vi "myo_test.vi"() -> ()   [LabVIEW 2013]
uses:
  <vilib>/BLE/type_def/connection_status_bundle.ctl
  <vilib>/BLE/type_def/address_type.ctl
  <vilib>/BLE/ble_functions/ble_write_by_service_characteristic_uint16.vi
panel:
  out "element":u8
  out "8bit integer 2":i8[][](array[numeric])
  out "8bit integer":u8[][](array[numeric])
  in  "Address Type":T1=1 items=["Public", "Random"]
  out "Readings":i32
  in  "stop":bool
  out "Handle table":string[][](array[string])
  out "Connection Status":T2={"MAC Address"="", "cnx handle"=0, "cnx flags"=0, "Address Type"=125, "Connection Interval (ms)"=125, "Timeout(ms)"=125, "Latency"=0, "bonding handle"=0} {"Address Type" items=["Public", "Random"]}
  out "Scanning":bool
  in  "Continue":bool
  in  "MAC Address":string
  in  "COM Bluegiga in":refnum<visa-resource-name>="COM13"
  out "Devices":string[][](array[string])
  out "BLED112 Dongle Info":string
  # "DISCOVER"
  # "CONNECT"
  # "Introduce the MAC Address of the device you want to connect and click in the CONTINUE button"
  # "READING"
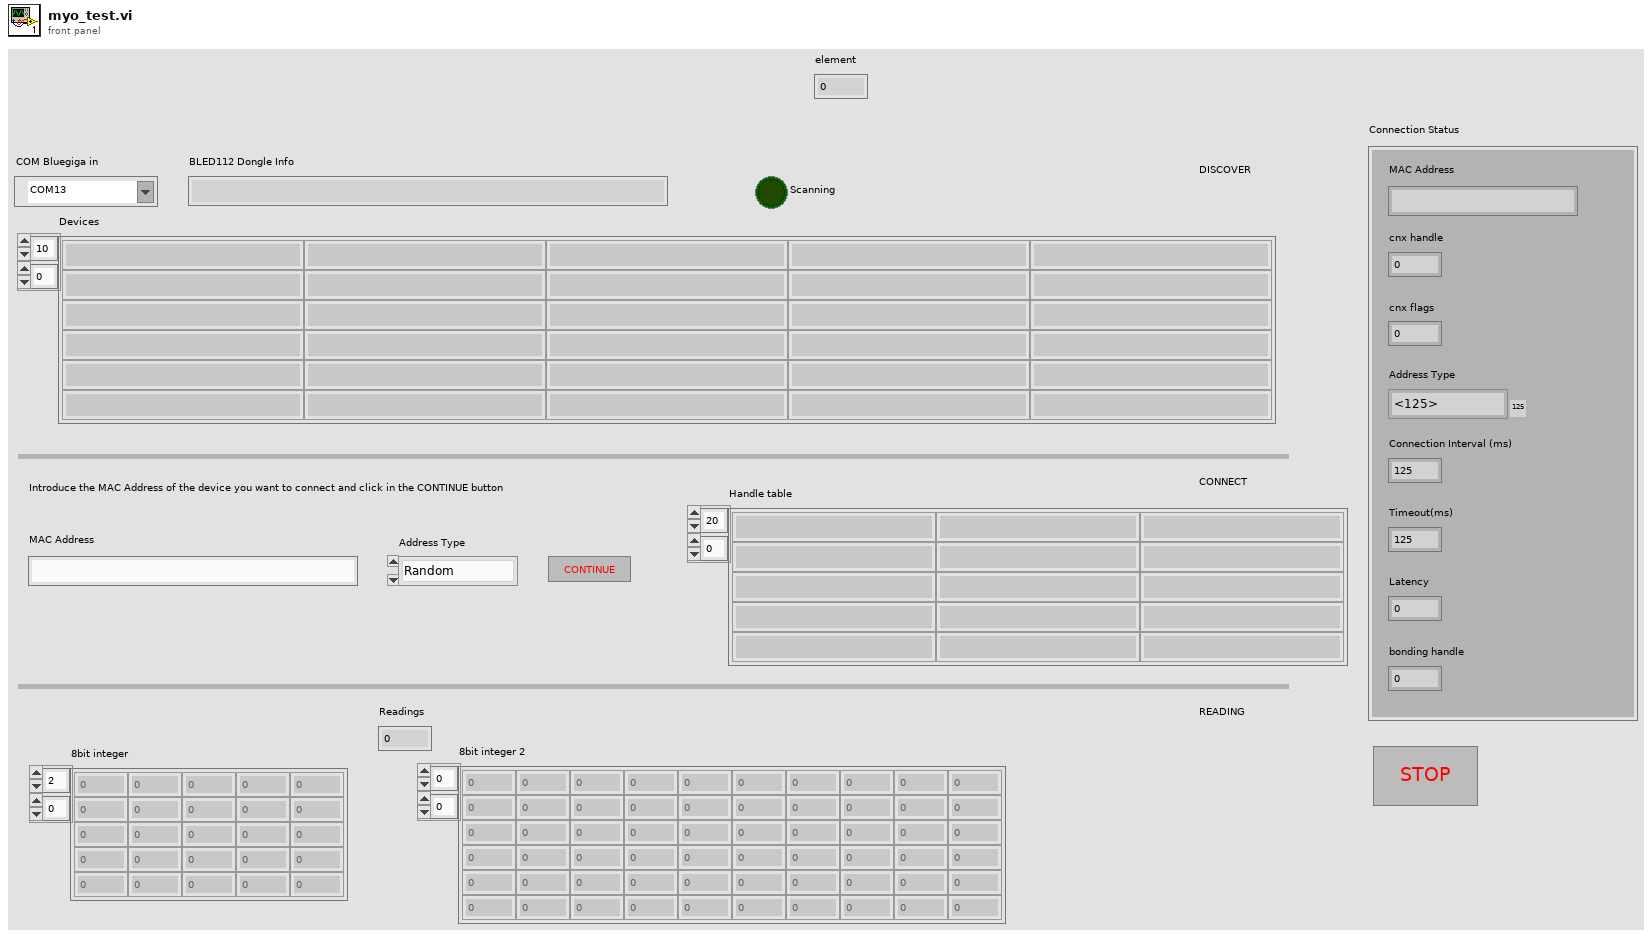
[diagram p1: front panel]
types:
  T1 = typedef "address_type.ctl" = u8
  T2 = typedef "connection_status_bundle.ctl" = cluster{"MAC Address":string, "cnx handle":u8, "cnx flags":u8, "Address Type":T1, "Connection Interval (ms)":u16, "Timeout(ms)":u16, "Latency":u16, "bonding handle":u8}
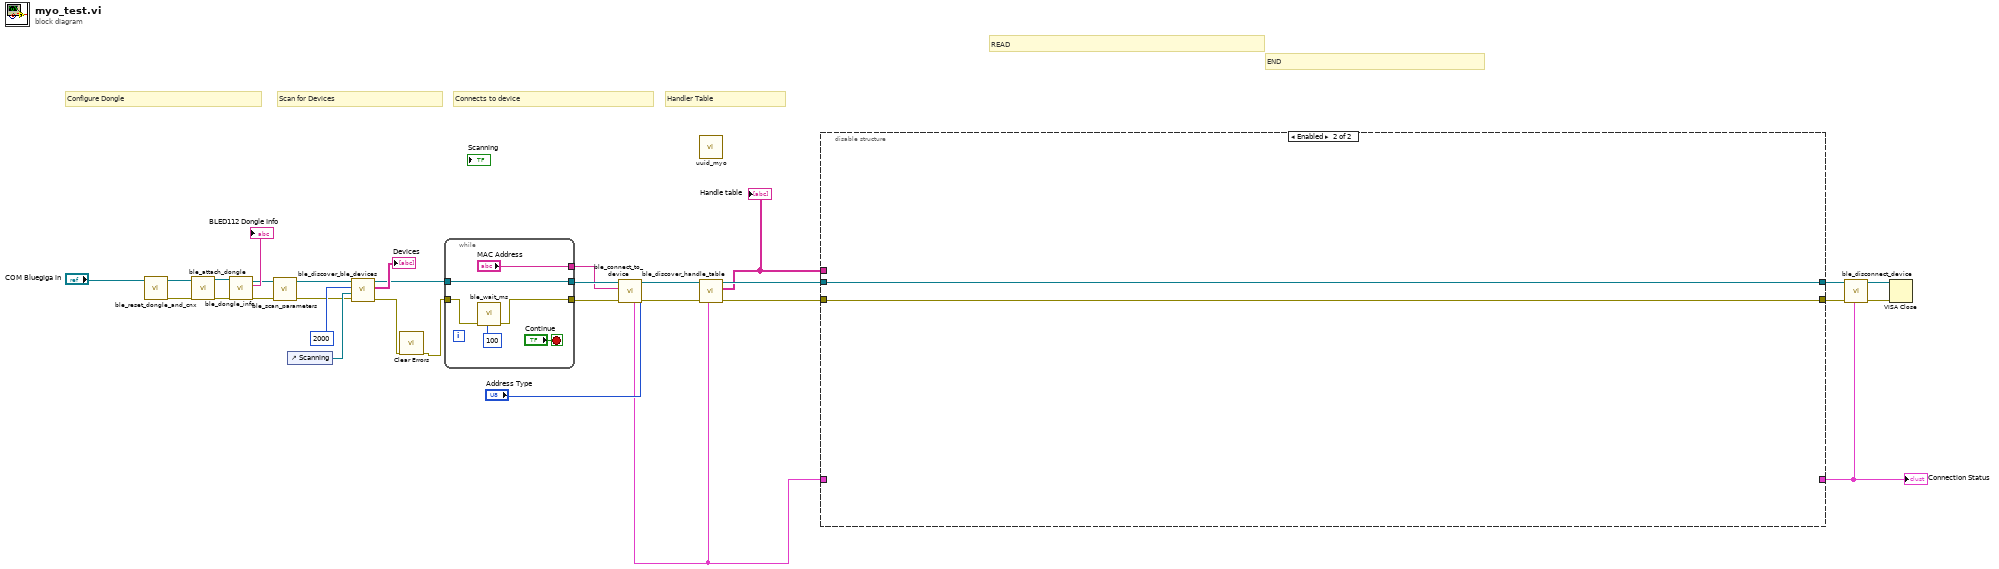
[diagram p0: block diagram]
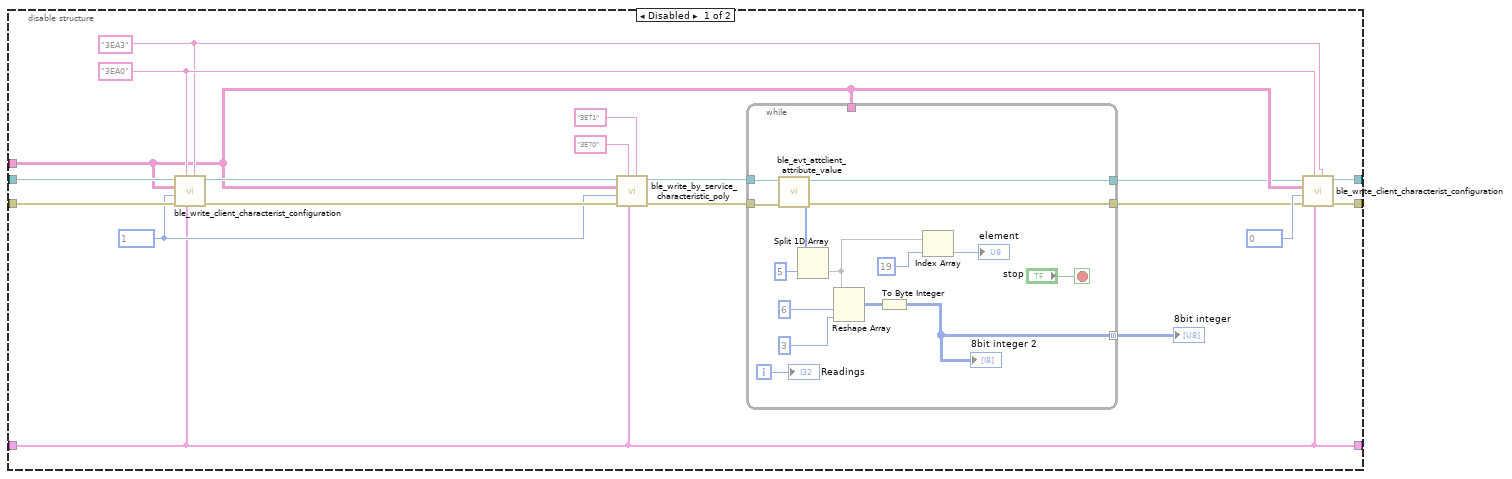
[diagram p2: hidden frame]
diagram:
  # "Handler Table"
  # "Connects to device"
  # "Scan for Devices"
  # "END"
  # "READ"
  # "Configure Dongle"
  n1 = call <vilib>:"ble_reset_dongle_and_cnx.vi"("COM Bluegiga in"="COM Bluegiga in") -> ("error out"=w15:errorcluster, "COM Bluegiga out"=w13:refnum<visa-resource-name>)  [unwired: 9 in]
  n2 = call <vilib>:"ble_attach_dongle.vi"("error in (no error)"=w15, "COM Bluegiga in"=w13) -> ("error out"=w17:errorcluster, "COM Bluegiga out"=w16:refnum<visa-resource-name>)  [unwired: 8 in]
  n3 = call <vilib>:"ble_dongle_info.vi"("error in (no error)"=w17, "COM Bluegiga in"=w16) -> ("error out"=w23:errorcluster, "info"=→"BLED112 Dongle Info":string, "COM Bluegiga out"=w24:refnum<visa-resource-name>)  [unwired: 7 in]
  n4 = call <vilib>:"ble_scan_parameters.vi"("error in (no error)"=w23, "COM Bluegiga in"=w24) -> ("error out"=w21:errorcluster, "COM Bluegiga out"=w22:refnum<visa-resource-name>)  [unwired: 7 in, 1 out]
  n5 = control-ref of="Scanning"() -> (w27:refnum<vi>)
  n6 = call <vilib>:"ble_discover_ble_devices.vi"("error in (no error)"=w21, "LED ref"=w27, "Scan Duration (10000ms)"=u32 2000, "COM Bluegiga in"=w22) -> ("error out"=w8:errorcluster, "Devices"=→"Devices":string[][], "COM Bluegiga out"=w28:refnum<visa-resource-name>)  [unwired: 5 in]
  n7 = call <vilib>:"Clear Errors.vi"("error in (no error)"=w8) -> ("error out"=w7:errorcluster)  [unwired: 6 in]
  n8 = while {
    tunnel: w7 -> [w36]
    tunnel: [w35] -> w26
    tunnel: w28 -> [w35]
    tunnel: [w34] -> w25
    tunnel: ["MAC Address"] -> w18
    stop <- "Continue" stop-if-true
    n9 = call <vilib>:"ble_wait_ms.vi"("milliseconds to wait (100)"=u32 100, "error in (no error)"=w36) -> ("error out"=w34:errorcluster)  [unwired: 9 in]
  }
  n10 = call <vilib>:"ble_connect_to_device.vi"("Address Type"="Address Type", "error in (no error)"=w25, "MAC Address"=w18, "COM Bluegiga in"=w26) -> ("error out"=w11:errorcluster, "COM Bluegiga out"=w12:refnum<visa-resource-name>, "Connection Status"=w2:T2)  [unwired: 5 in]
  n11 = call <vilib>:"ble_discover_handle_table.vi"("Connection Status"=w2, "error in (no error)"=w11, "COM Bluegiga in"=w12) -> ("error out"=w4:errorcluster, "Handle table"=w3:string[][], "COM Bluegiga out"=w5:refnum<visa-resource-name>)  [unwired: 6 in]
  "Handle table" <- w3
  n12 = call "uuid_myo.vi"() -> ()  [unwired: 11 in, 1 out]
  n13 = disable-structure shown="Enabled" {
    disable-tunnel: [w56 w72] -> w10
    disable-tunnel: [w55 w73] -> w9
    disable-tunnel: w5 -> [w51 w73]
    disable-tunnel: w4 -> [w50 w72]
    disable-tunnel: w3 -> [w44 _]
    disable-tunnel: w2 -> [w38 _]
    disable-tunnel: [w38 _] -> w1
    frame Disabled {
      w48 = u16 1 ("Value(16bit)")
      w54 = "3EA0" ("Service UUID")
      w53 = "3EA3" ("Characteristic UUID")
      n14 = call <vilib>:"ble_write_client_characterist_configuration.vi"("Characteristic UUID"=w53, "Connection Status"=w38, "Service UUID"=w54, "error in (no error)"=w50, "Value(16bit)"=w48, "Handle table"=w44, "COM Bluegiga in"=w51) -> ("error out"=w49:errorcluster, "COM Bluegiga out"=w45:refnum<visa-resource-name>)  [unwired: 3 in]
      n15 = call-poly <vilib>:"ble_write_by_service_characteristic_poly.vi"("Characteristic UUID"="3E71", "Connection Status"=w38, "Service UUID"="3E70", "error in (no error)"=w49, "Value(16bit)"=w48, "Handle table"=w44, "COM Bluegiga in"=w45) -> ("error out"=w43:errorcluster, "COM Bluegiga out"=w42:refnum<visa-resource-name>)  [unwired: 3 in]
      n16 = while {
        tunnel: w43 -> [w68]
        tunnel: w42 -> [w69]
        tunnel: w44 -> [_]
        tunnel: [w67] -> w41
        tunnel: [w66] -> w40
        tunnel: [w63] -> w39 mode=concatenating
        i -> [w70]
        stop <- "stop" stop-if-true
        n17 = call <vilib>:"ble_evt_attclient_attribute_value.vi"("error in (no error)"=w68, "COM Bluegiga in"=w69) -> ("error out"=w66:errorcluster, "characteristic value"=w61:u8[], "COM Bluegiga out"=w67:refnum<visa-resource-name>)  [unwired: 6 in, 1 out]
        n18 = Split 1D Array(array=w61, index=5) -> (second subarray=w59:u8[])  [unwired: 1 out]
        n19 = Reshape Array(w59, 6 ("dimension size"), 3 ("dimension size")) -> (w64:u8[][])
        n20 = To Byte Integer(number=w64) -> (8bit integer=w63:i8[][])
        "8bit integer 2" <- w63
        n21 = Index Array(array=w59, index=19) -> (element=→"element":u8)
        "Readings" <- w70
      }
      "8bit integer" <- w39
      n22 = call <vilib>:"ble_write_client_characterist_configuration.vi"("Characteristic UUID"=w53, "Connection Status"=w38, "Service UUID"=w54, "error in (no error)"=w40, "Value(16bit)"=u16 0, "Handle table"=w44, "COM Bluegiga in"=w41) -> ("error out"=w56:errorcluster, "COM Bluegiga out"=w55:refnum<visa-resource-name>)  [unwired: 3 in]
    }
    frame Enabled {
    }
  }
  "Connection Status" <- w1
  n23 = call <vilib>:"ble_disconnect_device.vi"("Connection Status"=w1, "error in (no error)"=w10, "COM Bluegiga in"=w9) -> ("error out"=w19:errorcluster, "COM Bluegiga out"=w20:refnum<visa-resource-name>)  [unwired: 7 in]
  n24 = VISA Close(VISA resource name=w20, error in (no error)=w19) -> ()  [unwired: 1 out]
